vi "destroy.vi"(8 "error in (no error)":errorcluster, 11 "ITaskStopMechanism in":refnum<class "ITaskStopMechanism.lvclass">) -> (0 "error out":errorcluster, 3 "ITaskStopMechanism out":refnum<class "ITaskStopMechanism.lvclass">)   [LabVIEW 2023, in "TLC_Daemon.lvlib" / "ITaskStopMechanism.lvclass"]
doc: "Destroy procedure"
uses:
  ITaskStopMechanism.lvclass
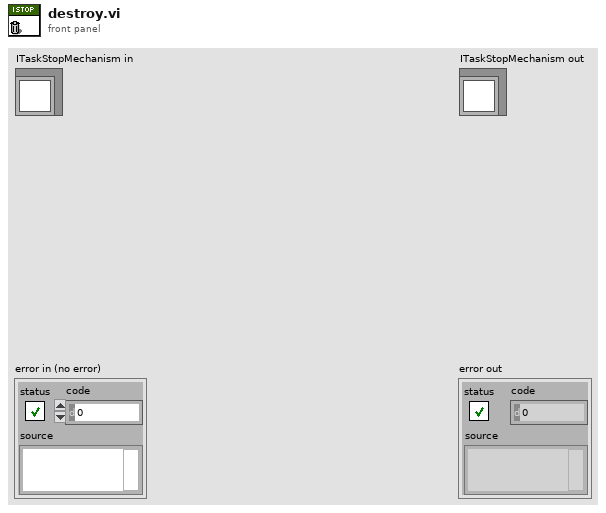
[diagram p1: front panel]
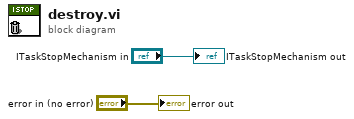
[diagram p0: block diagram]
diagram:
  "error out" <- "error in (no error)"
  "ITaskStopMechanism out" <- "ITaskStopMechanism in"
